vi "GV_Destructor.vi"(8 "error in (no error)":errorcluster, 11 "Gviewer in":refnum<class "Gviewer.lvclass">) -> (0 "error out":errorcluster, 3 "Gviewer out":refnum<class "Gviewer.lvclass">)   [LabVIEW 2020, in "Sgraph_lib_V1.lvlib" / "Gviewer.lvclass"]
doc: "Sgraph Gviewer destructor, close communication channel and unsubscribe from the server. Save current Viewer data if needed."
uses:
  Gviewer.lvclass
  Gviewer.lvclass/Gviewer.ctl
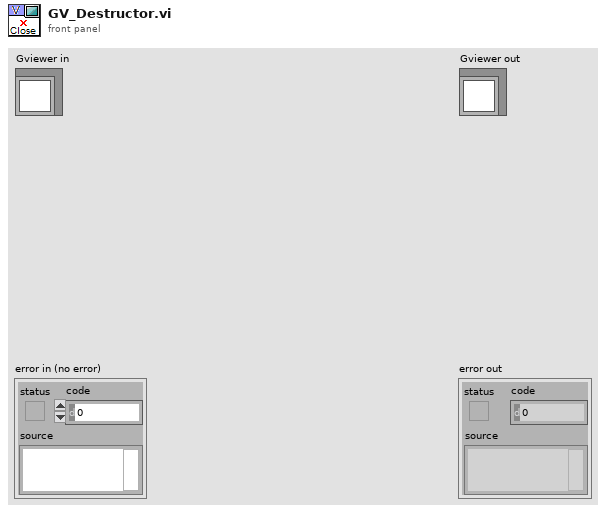
[diagram p1: front panel]
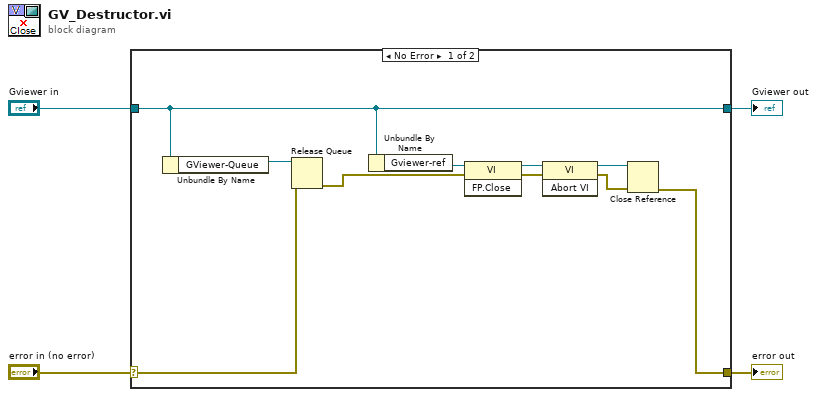
[diagram p0: block diagram]
diagram:
  n1 = case shown="No Error" "error in (no error)" {
    selector: "error in (no error)" -> [w13 w16]
    tunnel: [w5 w16] -> w3
    tunnel: [w12 w15] -> w1
    tunnel: "Gviewer in" -> [w12 w15]
    frame No Error {
      n2 = Unbundle By Name(w12) -> ("GViewer-Queue"=w14:refnum<queue>)
      n3 = Release Queue(queue=w14, error in (no error)=w13) -> (error out=w6:errorcluster)  [unwired: 1 in, 2 out]
      n4 = Unbundle By Name(w12) -> ("Gviewer-ref"=w11:refnum<vi>)
      n5 = invoke class="VI" method="FP.Close"(reference=w11, error in=w6) -> (reference out=w10:refnum<vi>, error out=w9:errorcluster)  [unwired: 1 in, 1 out]
      n6 = invoke class="VI" method="Abort VI"(reference=w10, error in=w9) -> (reference out=w8:refnum<vi>, error out=w7:errorcluster)  [unwired: 1 in, 1 out]
      n7 = Close Reference(reference=w8, error in (no error)=w7) -> (error out=w5:errorcluster)
    }
    frame Error {
    }
  }
  "error out" <- w3
  "Gviewer out" <- w1
